vi "Verify Credentials.vi"(4 "Access Token Secret (In)":string, 6 "Access Token (In)":string, 8 "error in (no error)":errorcluster, 10 "Consumer Secret":string, 11 "Consumer Key":string) -> (0 "error out":errorcluster, 1 "Screen Name":string, 2 "Success?":bool, 3 "HTTP Error Code":i32)   [LabVIEW 2011, in "i3-twitter.lvlib"]
doc: "Attempts to verify the supplied credentials with Twitter.com. If the credential are invalid, the user will be asked to enter his username and password.\n\nhttps://api.twitter.com/1/account/verify_credentials.xml"
uses:
  i3-twitter.lvlib
  i3-oauth/Controls/OAuth Credentials.ctl
  i3-oauth/Controls/Signature Method.ctl
  i3-oauth/Controls/HTTP Method.ctl
  <vilib>/httpClient/LabVIEWHTTPClient.lvlib
  i3-oauth/i3-oauth.lvlib
  i3-json/i3-json.lvlib
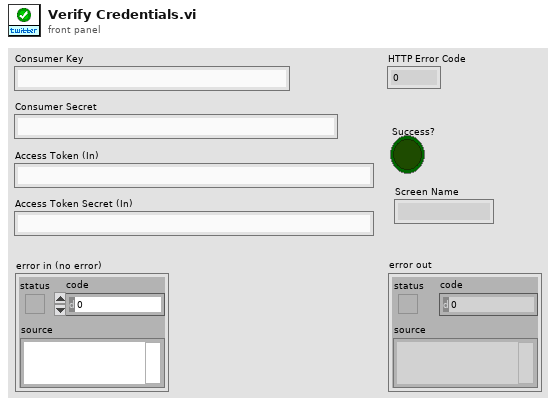
[diagram p1: front panel]
types:
  T1 = typedef "i3-oauth.lvlib/HTTP Method.ctl" = enum16{"GET", "POST", "PUT", "DELETE"}
  T2 = typedef "i3-oauth.lvlib/OAuth Credentials.ctl" = cluster{"Consumer Key":string, "Signature Method":T3, "Token":string, "Version":string, "Token Secret":string, "Consumer Secret":string}
  T3 = typedef "i3-oauth.lvlib/Signature Method.ctl" = enum16{"HMAC-MD5", "HMAC-SHA1", "HMAC-SHA224", "HMAC-SHA256", "HMAC-SHA384", "HMAC-SHA512"}
  T4 = typedef "LabVIEWHTTPClient.lvlib/ClientHandle.ctl" = refnum<k1>
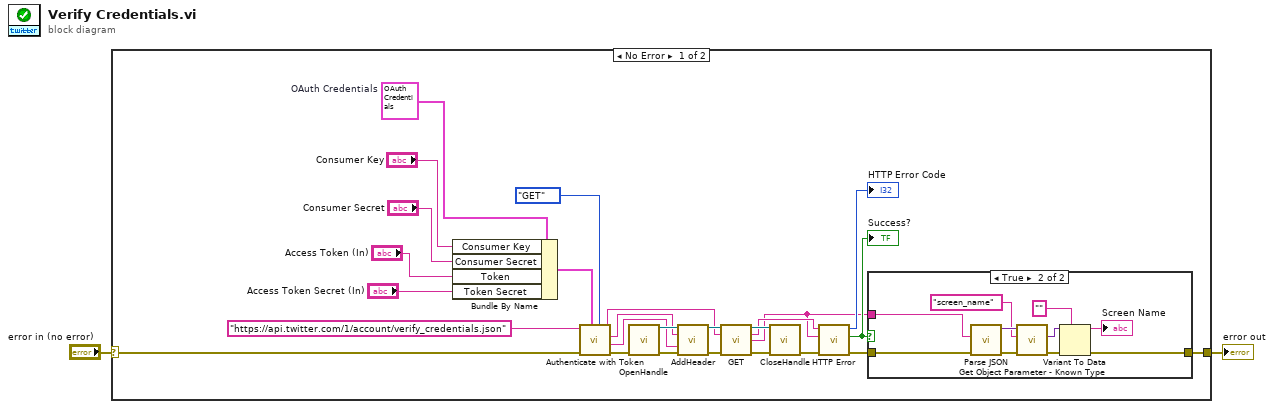
[diagram p0: block diagram]
diagram:
  n1 = case shown="No Error" "error in (no error)" {
    selector: "error in (no error)" -> [w4 w40]
    tunnel: [w9 w40] -> w2
    frame No Error {
      w26 = T2 {"Consumer Key"="", "Signature Method"=enum."HMAC-SHA1", "Token"="", "Version"="1.0", "Token Secret"="", "Consumer Secret"=""}  # OAuth Credentials
      n2 = Bundle By Name(cluster=w26, "Consumer Key"="Consumer Key", "Consumer Secret"="Consumer Secret", "Token"="Access Token (In)", "Token Secret"="Access Token Secret (In)") -> (w17:T2)
      n3 = call "Authenticate with Token.vi"("HTTP Method"=HTTP_Method."GET", "OAuth Credentials"=w17, "error in (no error)"=w4, "Base URL"="https://api.twitter.com/1/account/verify_credentials.json") -> ("error out"=w5:errorcluster, "Header Value"=w11:string, "Header Parameter"=w14:string, "Full URL"=w3:string)  [unwired: 3 in, 1 out]
      n4 = call <vilib>:"OpenHandle.vi"("error in (no error)"=w5) -> ("client handle out"=w15:T4, "error out"=w6:errorcluster)  [unwired: 13 in]
      n5 = call <vilib>:"AddHeader.vi"("client handle"=w15, "header"=w14, "value"=w11, "error in (no error)"=w6) -> ("client handle out"=w13:T4, "error out"=w16:errorcluster)  [unwired: 10 in]
      n6 = call <vilib>:"GET.vi"("client handle"=w13, "url"=w3, "error in (no error)"=w16) -> ("client handle out"=w27:T4, "headers"=w24:string, "body"=w7:string, "error out"=w28:errorcluster)  [unwired: 9 in]
      n7 = call <vilib>:"CloseHandle.vi"("client handle"=w27, "error in (no error)"=w28) -> ("error out"=w23:errorcluster)  [unwired: 13 in]
      n8 = call "HTTP Error.vi"("error in (no error)"=w23, "Body"=w7, "Header"=w24) -> ("error out"=w10:errorcluster, "Success?"=w8:bool, "HTTP Error Code"=→"HTTP Error Code":i32)  [unwired: 6 in]
      "Success?" <- w8
      n9 = case shown="True" w8 {
        tunnel: w7 -> [_ w39]
        tunnel: w10 -> [w29 w33]
        tunnel: [w29 w30] -> w9
        frame False {
        }
        frame True {
          n10 = call "Parse JSON.vi"("error in (no error)"=w33, "JSON String"=w39) -> ("error out"=w32:errorcluster, "JSON Tree"=w38:variant)  [unwired: 6 in, 2 out]
          n11 = call "Get Object Parameter - Known Type.vi"("error in (no error)"=w32, "Parameter Name"="screen_name", "JSON Tree In (JSON Object)"=w38) -> ("error out"=w31:errorcluster, "Value"=w35:variant)  [unwired: 3 in, 4 out]
          n12 = Variant To Data(error in=w31, type="" ("Parameter Name"), Variant=w35) -> (data=→"Screen Name":string, error out=w30:errorcluster)
        }
      }
    }
    frame Error {
    }
  }
  "error out" <- w2
